vi "Calculate.vi"(8 "error in (no error)":errorcluster, 9 "Reference Rectangle":T1, 10 "My VI":string, 11 "Auto-Stretch in":refnum<class "Auto-Stretch.lvclass">) -> (0 "error out":errorcluster, 1 "Height":i16, 2 "Width":i16)   [LabVIEW 2017, in "MGI-Panel Manager.lvlib" / "Auto-Stretch.lvclass"]
doc: "Determines the size of the window.\n\n----\nPlease see the following web address for additional documentation and tutorial information:\nhttp://www.mooregoodideas.com/mgi-panel-manager/\n\nAuthor: Derek Trepanier\n\nCopyright (c) 2018, Moore Good Ideas, Inc.\n\nAll rights reserved.\n\nRedistribution and use in source and binary forms, with or without modification, are permitted provided that the following conditions are met:\n\n * Redistributions of source code must retain the above copyright notice, this list of conditions and the following disclaimer.\n * Redistributions in binary form must reproduce the above copyright notice, this list of conditions and the following disclaimer in the documentation and/or other materials provided with the distribution.\n * Neither the name of Moore Good Ideas, Inc. nor the names of its contributors may be used to endorse or promote products derived from this software without specific prior written permission.\n\nTHIS SOFTWARE IS PROVIDED BY THE COPYRIGHT HOLDERS AND CONTRIBUTORS \"AS IS\" AND ANY EXPRESS OR IMPLIED WARRANTIES, INCLUDING, BUT NOT LIMITED TO, THE IMPLIED WARRANTIES OF MERCHANTABILITY AND FITNESS FOR A PARTICULAR PURPOSE ARE DISCLAIMED. IN NO EVENT SHALL THE COPYRIGHT OWNER OR CONTRIBUTORS BE LIABLE FOR ANY DIRECT, INDIRECT, INCIDENTAL, SPECIAL, EXEMPLARY, OR CONSEQUENTIAL DAMAGES (INCLUDING, BUT NOT LIMITED TO, PROCUREMENT OF SUBSTITUTE GOODS OR SERVICES; LOSS OF USE, DATA, OR PROFITS; OR BUSINESS INTERRUPTION) HOWEVER CAUSED AND ON ANY THEORY OF LIABILITY, WHETHER IN CONTRACT, STRICT LIABILITY, OR TORT (INCLUDING NEGLIGENCE OR OTHERWISE) ARISING IN ANY WAY OUT OF THE USE OF THIS SOFTWARE, EVEN IF ADVISED OF THE POSSIBILITY OF SUCH DAMAGE."
uses:
  Auto-Stretch.lvclass
  <vilib>/Utility/miscctls.llb/LVRectTypeDef.ctl
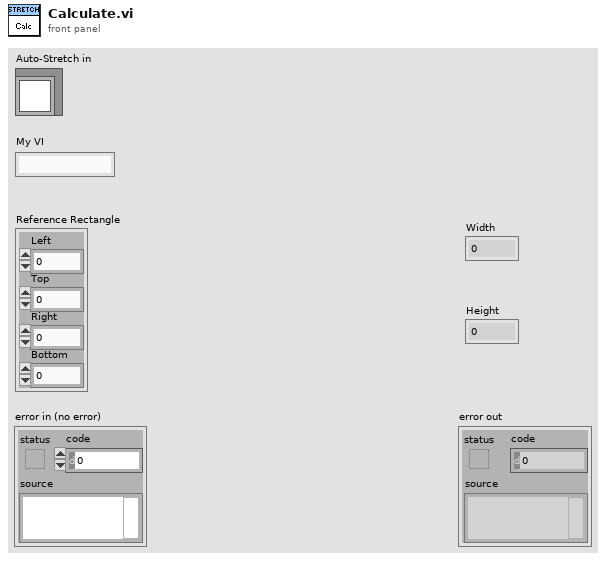
[diagram p1: front panel]
types:
  T1 = typedef "LVRectTypeDef.ctl" = cluster{"Left":i16, "Top":i16, "Right":i16, "Bottom":i16}
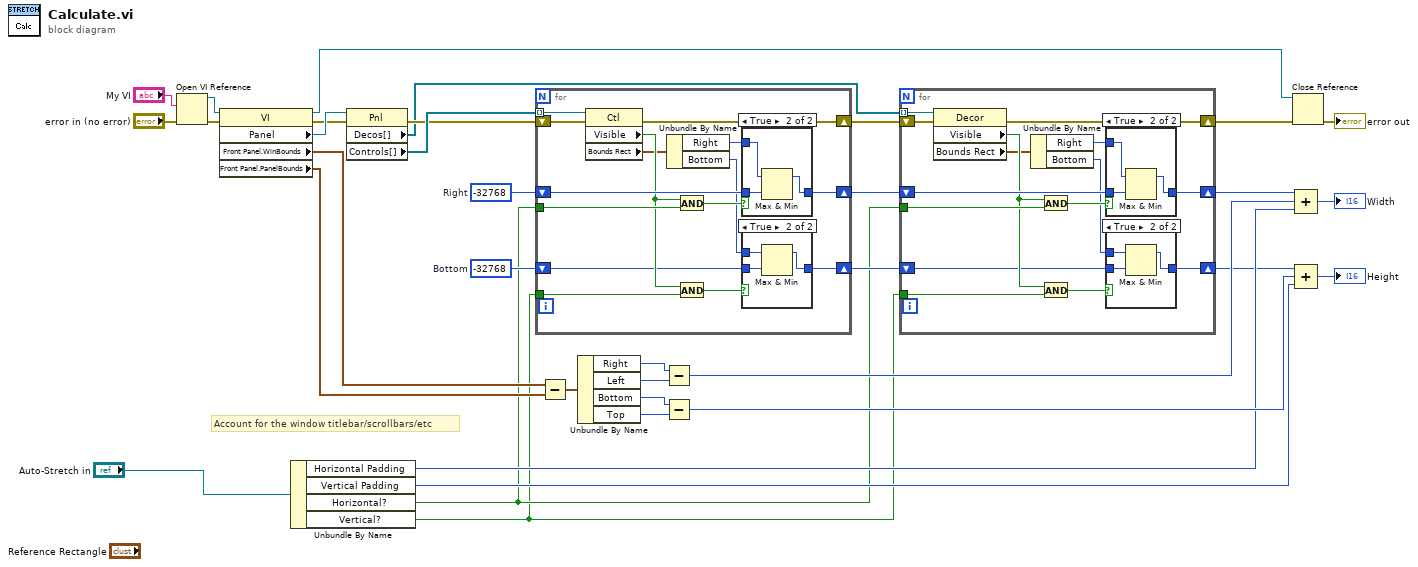
[diagram p0: block diagram]
diagram:
  w23 = i16 -32768  # Bottom
  w28 = i16 -32768  # Right
  # "Account for the window titlebar/scrollbars/etc"
  n1 = Open VI Reference(vi path="My VI", error in (no error)="error in (no error)") -> (vi reference=w33:refnum<vi>, error out=w32:errorcluster)  [unwired: 4 in]
  n2 = property class="VI"(reference=w33, error in=w32) -> (reference out=w25:refnum<vi>, error out=w30:errorcluster, "Panel"=w31:refnum<vi>, "Front Panel.WinBounds"=w20:T1, "Front Panel.PanelBounds"=w19:T1)
  n3 = Unbundle By Name("Auto-Stretch in") -> ("Horizontal Padding"=w11:i16, "Vertical Padding"=w10:i16, "Horizontal?"=w3:bool, "Vertical?"=w2:bool)
  n4 = property class="Pnl"(reference=w31, error in=w30) -> (error out=w26:errorcluster, "Decos[]"=w1:refnum<vi>[], "Controls[]"=w29:refnum<vi>[])  [unwired: 1 out]
  n5 = for {
    tunnel: w29 -> [w50] mode=indexing
    shift-right: [w48] -> w9
    shift-left: w28 -> [w49]
    tunnel: w3 -> [w46]
    tunnel: w2 -> [w44]
    shift-right: [w42] -> w8
    shift-left: w26 -> [w43]
    shift-right: [w41] -> w7
    shift-left: w23 -> [w39]
    n6 = property class="Ctl"(reference=w50, error in=w43) -> (error out=w42:errorcluster, "Visible"=w45:bool, "Bounds Rect"=w36:T1)  [unwired: 1 out]
    n7 = Unbundle By Name(w36) -> ("Right"=w38:i16, "Bottom"=w37:i16)
    n8 = And(x=w45, y=w46) -> (x .and. y?=w47:bool)
    n9 = And(x=w45, y=w44) -> (x .and. y?=w40:bool)
    n10 = case shown="True" w47 {
      tunnel: w49 -> [w55 w58]
      tunnel: [w55 w57] -> w48
      tunnel: w38 -> [_ w56]
      frame False {
      }
      frame True {
        n11 = Max & Min(x=w56, y=w58) -> (max(x,y)=w57:i16)  [unwired: 1 out]
      }
    }
    n12 = case shown="True" w40 {
      tunnel: w39 -> [w51 w54]
      tunnel: [w51 w53] -> w41
      tunnel: w37 -> [_ w52]
      frame False {
      }
      frame True {
        n13 = Max & Min(x=w52, y=w54) -> (max(x,y)=w53:i16)  [unwired: 1 out]
      }
    }
  }
  n14 = Subtract(x=w20, y=w19) -> (x-y=w14:T1)
  n15 = Unbundle By Name(w14) -> ("Right"=w18:i16, "Left"=w17:i16, "Bottom"=w16:i16, "Top"=w15:i16)
  n16 = Subtract(x=w18, y=w17) -> (x-y=w13:i16)
  n17 = Subtract(x=w16, y=w15) -> (x-y=w12:i16)
  n18 = for {
    tunnel: w1 -> [w73] mode=indexing
    shift-right: [w71] -> w5
    shift-left: w9 -> [w72]
    tunnel: w3 -> [w69]
    tunnel: w2 -> [w67]
    shift-right: [w65] -> w6
    shift-left: w8 -> [w66]
    shift-right: [w64] -> w4
    shift-left: w7 -> [w62]
    n19 = property class="Decor"(reference=w73, error in=w66) -> (error out=w65:errorcluster, "Visible"=w68:bool, "Bounds Rect"=w59:T1)  [unwired: 1 out]
    n20 = Unbundle By Name(w59) -> ("Right"=w61:i16, "Bottom"=w60:i16)
    n21 = And(x=w68, y=w69) -> (x .and. y?=w70:bool)
    n22 = And(x=w68, y=w67) -> (x .and. y?=w63:bool)
    n23 = case shown="True" w70 {
      tunnel: w72 -> [w78 w81]
      tunnel: [w78 w80] -> w71
      tunnel: w61 -> [_ w79]
      frame False {
      }
      frame True {
        n24 = Max & Min(x=w79, y=w81) -> (max(x,y)=w80:i16)  [unwired: 1 out]
      }
    }
    n25 = case shown="True" w63 {
      tunnel: w62 -> [w74 w77]
      tunnel: [w74 w76] -> w64
      tunnel: w60 -> [_ w75]
      frame False {
      }
      frame True {
        n26 = Max & Min(x=w75, y=w77) -> (max(x,y)=w76:i16)  [unwired: 1 out]
      }
    }
  }
  n27 = Close Reference(reference=w25, error in (no error)=w6) -> (error out=→"error out":errorcluster)
  n28 = Compound Arithmetic op=ADD(w5, w13, w11) -> (→"Width":i16)
  n29 = Compound Arithmetic op=ADD(w4, w12, w10) -> (→"Height":i16)
